vi "Test U16 Logic.vi"() -> ()   [LabVIEW 2021]
uses:
  Source/Abs_Types/U16 Integer/Simple Read.vi
  Source/Constants/Support/U16/Const_U16.lvclass
  C:/TSA/LV_Abstract/Source/Abs_Types/U16 Integer/Abs_U16 Integer.lvclass
  Source/Constants/Support/U16/U16.vi
  Source/Functions/Logic/Support/NOT/U16/Method.vi
  Source/Functions/Logic/Support/EXOR/U16/Method_Const.vi
  Source/Functions/Logic/Support/EXNOR/U16/Method_Const.vi
  Source/Functions/Logic/Support/NOR/U16/Method_Const.vi
  Source/Functions/Logic/Support/OR/U16/Method_Const.vi
  Source/Functions/Logic/Support/AND/U16/Method_Const.vi
  Source/Abs_Types/U16 Integer/Abs_U16 Integer.lvclass
  Source/Functions/Logic/Support/NOT/U16/NOT_U16.lvclass
  C:/TSA/LV_Abstract/Source/Abs_Types/Integer/Abs_Integer.lvclass
  C:/Program Files (x86)/National Instruments/LabVIEW 2021/vi.lib/TSA/Abstract Data Classes/Abs_Types/Numeric/Abs_Numeric.lvclass
  C:/Program Files (x86)/National Instruments/LabVIEW 2021/vi.lib/TSA/Abstract Data Classes/Abs_Types/Value/Abs_Value.lvclass
  C:/Program Files (x86)/National Instruments/LabVIEW 2021/vi.lib/TSA/Abstract Data Classes/Abs_Types/Type/Abs_Type.lvclass
  C:/TSA/LV_Abstract/Source/Constants/Support/U16/Const_U16.lvclass
  Source/Functions/Logic/Support/AND/U16/AND_U16.lvclass
  Source/Functions/Logic/Support/OR/U16/OR_U16.lvclass
  Source/Functions/Logic/Support/EXOR/U16/EXOR_U16.lvclass
  Source/Functions/Logic/Support/NOR/U16/NOR_U16.lvclass
  Source/Functions/Logic/Support/EXNOR/U16/EXNOR_U16.lvclass
panel:
  out "EXNOR":u16 format="%08b"
  out "NOR":u16 format="%08b"
  out "OR":u16 format="%08b"
  out "AND":u16 format="%08b"
  out "EXOR":u16 format="%08b"
  in  "Numeric 2":u16 format="%08b"
  in  "Numeric":u16 format="%08b"
  out "Not":u16 format="%08b"
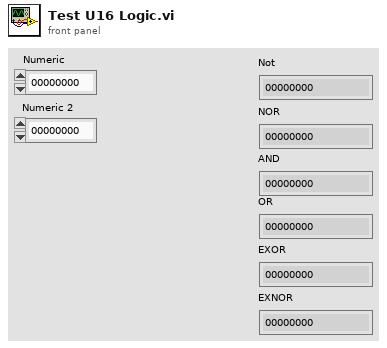
[diagram p1: front panel]
types:
  T1 = typedef "NOT_U16.lvclass/Abs_Type.ctl" = refnum<class "Abs_U16 Integer.lvclass">
  T2 = typedef "EXNOR_U16.lvclass/Abs_Type.ctl" = refnum<class "Abs_U16 Integer.lvclass">
  T3 = typedef "EXOR_U16.lvclass/Abs_Type.ctl" = refnum<class "Abs_U16 Integer.lvclass">
  T4 = typedef "NOR_U16.lvclass/Abs_Type.ctl" = refnum<class "Abs_U16 Integer.lvclass">
  T5 = typedef "OR_U16.lvclass/Abs_Type.ctl" = refnum<class "Abs_U16 Integer.lvclass">
  T6 = typedef "AND_U16.lvclass/Abs_Type.ctl" = refnum<class "Abs_U16 Integer.lvclass">
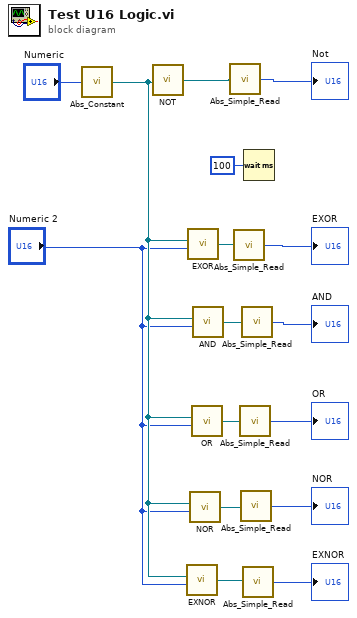
[diagram p0: block diagram]
diagram:
  n1 = call-poly "Abs_Constant.vi"("Value"="Numeric") -> ("Constant"=w15:refnum<class "Const_U16.lvclass">)  [unwired: 4 in]
  n2 = call-poly "NOT.vi"("Bool"=w15) -> ("Result"=w13:T1)  [unwired: 4 in]
  n3 = call-poly "EXNOR.vi"("Value"="Numeric 2", "A"=w15) -> ("Result"=w6:T2)  [unwired: 4 in]
  n4 = call-poly "EXOR.vi"("Value"="Numeric 2", "A"=w15) -> ("Result"=w11:T3)  [unwired: 4 in]
  n5 = call-poly "NOR.vi"("Value"="Numeric 2", "A"=w15) -> ("Result"=w7:T4)  [unwired: 4 in]
  n6 = call-poly "OR.vi"("Value"="Numeric 2", "A"=w15) -> ("Result"=w8:T5)  [unwired: 4 in]
  n7 = call-poly "AND.vi"("Value"="Numeric 2", "A"=w15) -> ("Result"=w9:T6)  [unwired: 4 in]
  n8 = call-poly "Abs_Simple_Read.vi"("Class"=w13) -> ("Value"=→"Not":u16)  [unwired: 4 in]
  n9 = call-poly "Abs_Simple_Read.vi"("Class"=w11) -> ("Value"=→"EXOR":u16)  [unwired: 4 in]
  n10 = call-poly "Abs_Simple_Read.vi"("Class"=w8) -> ("Value"=→"OR":u16)  [unwired: 4 in]
  n11 = call-poly "Abs_Simple_Read.vi"("Class"=w7) -> ("Value"=→"NOR":u16)  [unwired: 4 in]
  n12 = call-poly "Abs_Simple_Read.vi"("Class"=w9) -> ("Value"=→"AND":u16)  [unwired: 4 in]
  n13 = call-poly "Abs_Simple_Read.vi"("Class"=w6) -> ("Value"=→"EXNOR":u16)  [unwired: 4 in]
  n14 = Wait (ms)(milliseconds to wait=u32 100) -> ()  [unwired: 1 out]
